vi "WM Bretschneider.vi"(0 "Significant Wave Height":dbl=1.0 min=0.0 step=0.01 format="%.2f", 1 "Start Freq":dbl format="%.3f", 2 "Peak Wave Period":dbl=1.0 min=0.0 step=0.01 format="%.2f", 3 "Number of Frequencies":i32=100 min=1 step=1, 4 "End Freq":dbl=5.0 min=0.0 step=0.01 format="%.2f", 5 "Scale Ratio":dbl=1.0 min=0.0 step=0.01 format="%.2f") -> (6 "Spectral Energy":dbl[](array[numeric]) format="%.3p", 7 "Frequency":dbl[](array[numeric]) format="%.2f", 8 "Bretschneider parameters":T1 {"Scale Ratio" format="%.2f"; "Sig Wave Period" format="%.2f"; "Sig Wave Height" format="%.2f"})   [LabVIEW 2012]
panel:
  in  "Boolean":bool
  # "Bretschneider Wave Spectra"
  # "m"
  # "(Full Scale)"
  # "s"
  # "(Full Scale)"
  # ":1"
  # "Full Scale : Model Scale"
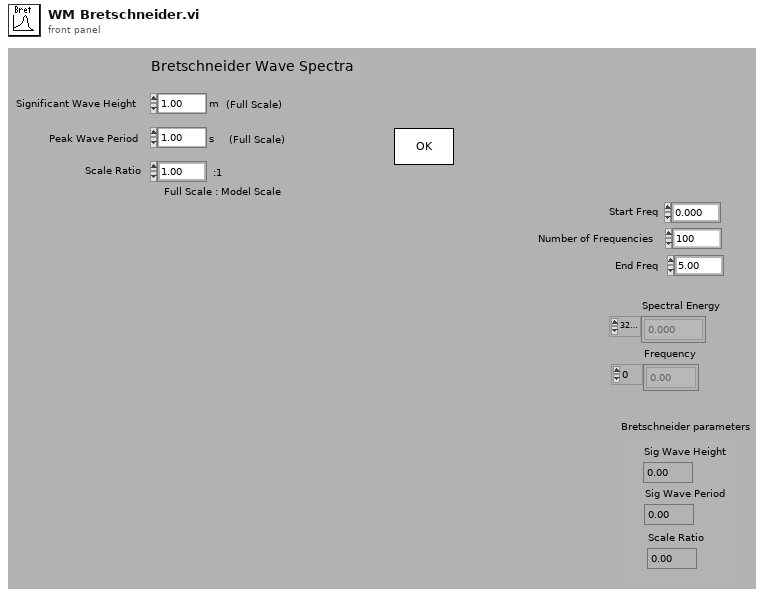
[diagram p1: front panel]
types:
  T1 = cluster{"Sig Wave Height":dbl, "Sig Wave Period":dbl, "Scale Ratio":dbl}
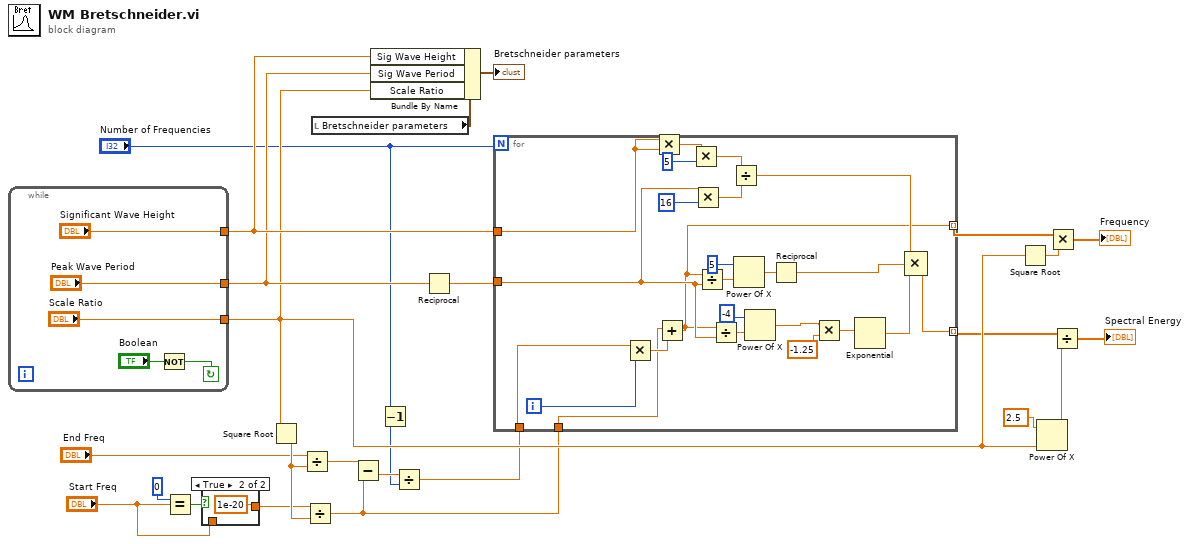
[diagram p0: block diagram]
diagram:
  n1 = while {
    tunnel: ["Scale Ratio"] -> w21
    tunnel: ["Peak Wave Period"] -> w22
    tunnel: ["Significant Wave Height"] -> w23
    stop <- w26 continue-if-true
    n2 = Not(x="Boolean") -> (.not. x?=w26:bool)
  }
  n3 = Equal?(x=0, y="Start Freq") -> (x = y?=w8:bool)
  n4 = case shown="True" w8 {
    tunnel: [w31 1e-20] -> w2
    tunnel: "Start Freq" -> [w31 _]
    frame False {
    }
    frame True {
    }
  }
  n5 = Square Root(x=w21) -> (sqrt(x)=w6:dbl)
  n6 = Divide(x="End Freq", y=w6) -> (x/y=w7:dbl)
  n7 = Divide(x=w2, y=w6) -> (x/y=w5:dbl)
  n8 = local read "Bretschneider parameters"() -> (w24:T1)
  n9 = Subtract(x=w7, y=w5) -> (x-y=w20:dbl)
  n10 = Bundle By Name(cluster=w24, "Sig Wave Height"=w23, "Sig Wave Period"=w22, "Scale Ratio"=w21) -> (→"Bretschneider parameters":T1)
  n11 = Decrement(x="Number of Frequencies") -> (x-1=w18:i32)
  n12 = Divide(x=w20, y=w18) -> (x/y=w16:dbl)
  n13 = Reciprocal(x=w22) -> (1/x=w17:dbl)
  n14 = for {
    N: "Number of Frequencies" -> [_]
    tunnel: w23 -> [w40]
    tunnel: w17 -> [w39]
    tunnel: w5 -> [w36]
    tunnel: w16 -> [w34]
    tunnel: [w38] -> w11 mode=indexing
    tunnel: [w37] -> w14 mode=indexing
    i -> [w35]
    n15 = Multiply(x=w34, y=w35) -> (x*y=w41:dbl)
    n16 = Multiply(x=w40, y=w40) -> (x*y=w42:dbl)
    n17 = Add(x=w36, y=w41) -> (x+y=w38:dbl)
    n18 = Multiply(x=w42, y=i16 5) -> (x*y=w44:dbl)
    n19 = Multiply(x=w39, y=i16 16) -> (x*y=w43:dbl)
    n20 = Divide(x=w38, y=w39) -> (x/y=w47:dbl)
    n21 = Divide(x=w38, y=w39) -> (x/y=w50:dbl)
    n22 = Divide(x=w44, y=w43) -> (x/y=w54:dbl)
    n23 = Power Of X(1:w47, 2:i16 5 ("y")) -> (0:w49:dbl)
    n24 = Power Of X(1:w50, 2:i16 -4 ("y")) -> (0:w33:dbl)
    n25 = Reciprocal(x=w49) -> (1/x=w55:dbl)
    n26 = Multiply(x=w33, y=sgl -1.25) -> (x*y=w53:dbl)
    n27 = Exponential(1:w53) -> (0:w56:dbl)
    n28 = Compound Arithmetic op=MULTIPLY(w54, w55, w56) -> (w37:dbl)
  }
  n29 = Square Root(x=w21) -> (sqrt(x)=w10:dbl)
  n30 = Power Of X(1:w21, 2:2.5 ("y")) -> (0:w13:dbl)
  n31 = Multiply(x=w11, y=w10) -> (x*y=→"Frequency":dbl[])
  n32 = Divide(x=w14, y=w13) -> (x/y=→"Spectral Energy":dbl[])
